vi "Image.vi"(2 "XRef":refnum<vi>, 3 "State In":T1) -> (0 "Image":picture)   [LabVIEW 2012, in "Array Size Unbundle.xnode"]
uses:
  Array Size Unbundle.xnode
  State.ctl
  <vilib>/picture/picture.llb/imagedata.ctl
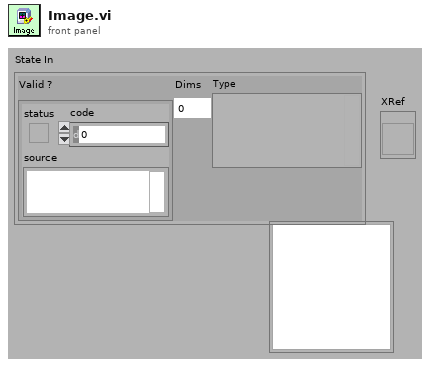
[diagram p1: front panel]
types:
  T1 = typedef "Array Size Unbundle.xnode/State.ctl" = cluster{"Valid ?":errorcluster, "Dims":i32, "Type":variant}
  T2 = typedef "imagedata.ctl" = cluster{"image type":i32, "image depth":i32, "image":u8[], "mask":u8[], "colors":u32[], "Rectangle":cluster{"left":i16, "top":i16, "right":i16, "bottom":i16}}
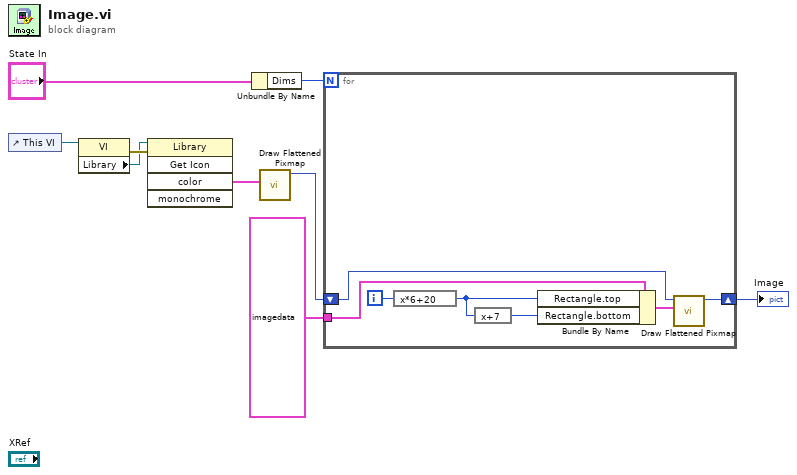
[diagram p0: block diagram]
diagram:
  n1 = control-ref of="This VI"() -> (w9:refnum<vi>)
  n2 = property class="VI"(reference=w9) -> (error out=w8:errorcluster, "Library"=w7:refnum<vi>)  [unwired: 1 in, 1 out]
  n3 = invoke class="Library" method="Get Icon"(reference=w7, error in=w8) -> ("color"=w6:T2)  [unwired: 3 in, 4 out]
  n4 = Unbundle By Name("State In") -> ("Dims"=w1:i32)
  n5 = call <vilib>:"Draw Flattened Pixmap.vi"("image data"=w6) -> ("new picture"=w3:picture)  [unwired: 1 in, 7 out]
  n6 = for {
    N: w1 -> [_]
    shift-right: [w15] -> w2
    shift-left: w3 -> [w16]
    tunnel: T2 {"image type"=0, "image depth"=24, "image"=[0, 0, 0, 248, 152, 48, 248, 152, 48, 248, 152, 48, 248, 152, 48, 248, 152, 48, 248, 152, 48, 248, 152, 48, 248, 152, 48, 248, 152, 48, 248, 152, 48, 248, 152, 48, 248, 152, 48, 248, 152, 48, 248, 152, 48, 248, 152, 48, 248, 152, 48, 248, 152, 48, 248, 152, 48, 248, 152, 48, 0, 0, 0, 0, 0, 0, 0, 0, 0, 0, 0, 0, 0, 0, 0, 248, 152, 48, 248, 152, 48, 248, 152, 48, 248, 152, 48, 248, 152, 48, 248, 152, 48, 0, 0, 0, 0, 0, 0, 248, 152, 48, 248, 152, 48, 248, 152, 48, 248, 152, 48, 248, 152, 48, 248, 152, 48, 248, 152, 48, 248, 152, 48, 248, 152, 48, 248, 152, 48, 248, 152, 48, 248, 152, 48, 248, 152, 48, 248, 152, 48, 248, 152, 48, 248, 152, 48, 248, 152, 48, 248, 152, 48, 248, 152, 48, 0, 0, 0, 248, 152, 48, 248, 152, 48, 248, 152, 48, 0, 0, 0, 248, 152, 48, 248, 152, 48, 248, 152, 48, 248, 152, 48, 248, 152, 48, 248, 152, 48, 0, 0, 0, 0, 0, 0, 248, 152, 48, 248, 152, 48, 248, 152, 48, 248, 152, 48, 248, 152, 48, 248, 152, 48, 248, 152, 48, 248, 152, 48, 248, 152, 48, 248, 152, 48, 248, 152, 48, 248, 152, 48, 248, 152, 48, 248, 152, 48, 248, 152, 48, 248, 152, 48, 248, 152, 48, 248, 152, 48, 248, 152, 48, 0, 0, 0, 248, 152, 48, 248, 152, 48, 248, 152, 48, 0, 0, 0, 248, 152, 48, 248, 152, 48, 248, 152, 48, 248, 152, 48, 248, 152, 48, 248, 152, 48, 0, 0, 0, 0, 0, 0, 248, 152, 48, 248, 152, 48, 248, 152, 48, 248, 152, 48, 248, 152, 48, 248, 152, 48, 248, 152, 48, 248, 152, 48, 248, 152, 48, 248, 152, 48, 248, 152, 48, 248, 152, 48, 248, 152, 48, 248, 152, 48, 248, 152, 48, 248, 152, 48, 248, 152, 48, 248, 152, 48, 248, 152, 48, 0, 0, 0, 248, 152, 48, 248, 152, 48, 248, 152, 48, 0, 0, 0, 248, 152, 48, 248, 152, 48, 248, 152, 48, 248, 152, 48, 248, 152, 48, 248, 152, 48, 0, 0, 0, 0, 0, 0, 248, 152, 48, 248, 152, 48, 248, 152, 48, 248, 152, 48, 248, 152, 48, 248, 152, 48, 248, 152, 48, 248, 152, 48, 248, 152, 48, 248, 152, 48, 248, 152, 48, 248, 152, 48, 248, 152, 48, 248, 152, 48, 248, 152, 48, 248, 152, 48, 248, 152, 48, 248, 152, 48, 248, 152, 48, 0, 0, 0, 0, 0, 0, 0, 0, 0, 0, 0, 0, 0, 0, 0, 248, 152, 48, 248, 152, 48, 248, 152, 48, 248, 152, 48, 248, 152, 48, 248, 152, 48, 0, 0, 0, 0, 0, 0, 248, 152, 48, 248, 152, 48, 248, 152, 48, 248, 152, 48, 248, 152, 48, 248, 152, 48, 248, 152, 48, 248, 152, 48, 248, 152, 48, 248, 152, 48, 248, 152, 48, 248, 152, 48, 248, 152, 48, 248, 152, 48, 248, 152, 48, 248, 152, 48, 248, 152, 48, 248, 152, 48, 248, 152, 48, 248, 152, 48, 248, 152, 48, 248, 152, 48, 248, 152, 48, 248, 152, 48, 248, 152, 48, 248, 152, 48, 248, 152, 48, 248, 152, 48, 248, 152, 48, 248, 152, 48, 0, 0, 0, 0, 0, 0, 0, 0, 0, 0, 0, 0, 0, 0, 0, 0, 0, 0, 0, 0, 0, 0, 0, 0, 0, 0, 0, 0, 0, 0, 0, 0, 0, 0, 0, 0, 0, 0, 0, 0, 0, 0, 0, 0, 0, 0, 0, 0, 0, 0, 0, 0, 0, 0, 0, 0, 0, 0, 0, 0, 0, 0, 0, 0, 0, 0, 0, 0, 0, 0, 0, 0, 0, 0, 0, 0, 0, 0, 0, 0, 0, 0, 0, 0, 0, 0, 0, 0, 0, 0, 0, 0, 0, 0, 0, 0, 0, 0, 0], "mask"=[], "colors"=[], "Rectangle"={"left"=0, "top"=0, "right"=32, "bottom"=7}} ("image data") -> [w14]
    i -> [w12]
    n7 = expression code="x*6+20"(w12) -> (w11:i32)
    n8 = expression code="x+7"(w11) -> (w10:i32)
    n9 = Bundle By Name(cluster=w14, "Rectangle.top"=w11, "Rectangle.bottom"=w10) -> (w13:T2)
    n10 = call <vilib>:"Draw Flattened Pixmap.vi"("image data"=w13, "picture"=w16) -> ("new picture"=w15:picture)  [unwired: 7 out]
  }
  "Image" <- w2
